vi "Students T Probability Distribution Function.vi"(10 "degrees of freedom":i32=1 min=1 format="%0.0f", 11 "( 1 - a )":dbl) -> (3 "Two-Sided":dbl format="%0.4f")   [LabVIEW 2017]
uses:
  <vilib>/gmath/statdist.llb/Student t Inverse CDF.vi
  <vilib>/gmath/NI_Gmath.lvlib
panel:
  out "( a / 2)":dbl
  out "( a )":dbl
  out "error":i32
  out "One-Sided":dbl format="%0.4f"
  # "(1-a) = probability that value is equal to the mean\n a = probability of exceeding the mean value for a one-sided test\na/2 = probability of exceeding (or being less than) the mean value for a TWO-sided test"
  # "Must be\n 0<(1-a)<1"
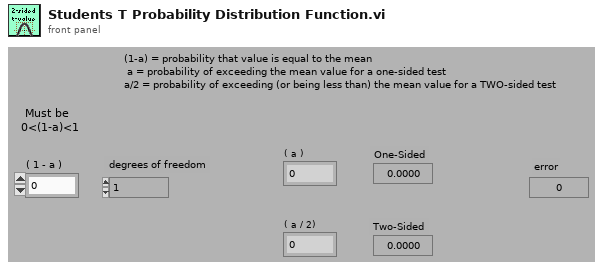
[diagram p1: front panel]
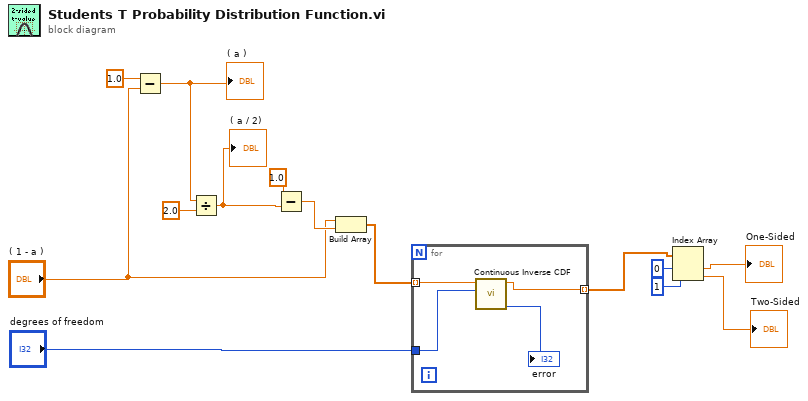
[diagram p0: block diagram]
diagram:
  n1 = Subtract(x=1.0, y="( 1 - a )") -> (x-y=w11:dbl)
  "( a )" <- w11
  n2 = Divide(x=w11, y=2.0) -> (x/y=w9:dbl)
  "( a / 2)" <- w9
  n3 = Subtract(x=1.0, y=w9) -> (x-y=w8:dbl)
  n4 = Build Array("( 1 - a )", w8) -> (w6:dbl[])
  n5 = for {
    tunnel: "degrees of freedom" -> [w16]
    tunnel: [w17] -> w5 mode=indexing
    tunnel: w6 -> [w18] mode=indexing
    n6 = call-poly <vilib>:"Continuous Inverse CDF.vi"("k degrees of freedom"=w16, "cdf(x)"=w18) -> ("error"=→"error":i32, "x"=w17:dbl)  [unwired: 8 in]
  }
  n7 = Index Array(array=w5, index #1=0 ("index"), index #2=1 ("index")) -> (element #1=→"One-Sided":dbl, element #2=→"Two-Sided":dbl)
